vi "CommitTransaction.vi"(8 "ErrorIn":errorcluster caption="Error In(no Error)", 9 "NIGUID":string, 11 "ReferenceIn":refnum<class "ErrorDefinitionSQLite.lvclass"> caption="Reference In") -> (0 "ErrorOut":errorcluster caption="Error Out", 3 "ReferenceOut":refnum<class "ErrorDefinitionSQLite.lvclass"> caption="Reference Out")   [LabVIEW 2021, in "ErrorDefinitionSQLite.lvclass"]
uses:
  ErrorDefinitionSQLite.lvclass
  <vilib>/drjdpowell/SQLite Library/Transaction Helpers/Transaction.lvlib
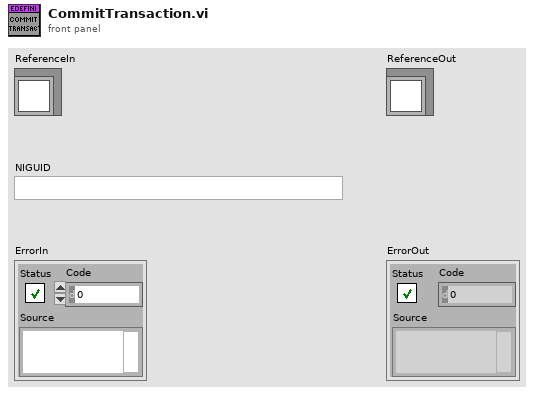
[diagram p1: front panel]
types:
  T1 = typedef "ErrorDefinitionSQLite.lvclass/ObjectAttributes.ctl" = cluster{"Path":path, "SQLiteRef":refnum<class "Connection.lvclass">, "EndOfRange":i32, "StartOfRange":i32}
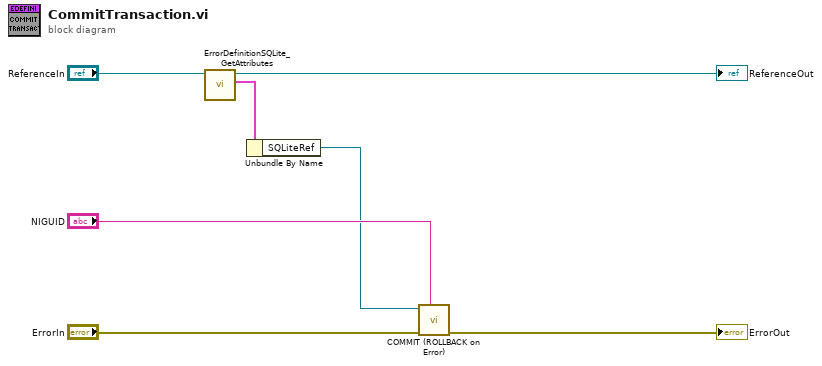
[diagram p0: block diagram]
diagram:
  n1 = call "ErrorDefinitionSQLite_GetAttributes.vi"("ReferenceIn"="ReferenceIn") -> ("Data"=w2:T1, "ReferenceOut"=→"ReferenceOut":refnum<class "ErrorDefinitionSQLite.lvclass">)  [unwired: 7 in, 2 out]
  n2 = Unbundle By Name(w2) -> ("SQLiteRef"=w1:refnum<class "Connection.lvclass">)
  n3 = call <vilib>:"COMMIT (ROLLBACK on Error).vi"("Savepoint name"="NIGUID", "error in (no error)"="ErrorIn", "SQLite Connection in"=w1) -> ("error out"=→"ErrorOut":errorcluster)  [unwired: 7 in, 1 out]
